vi "Read_MNK_Temperature.vi"(8 "Error in (no error)":errorcluster) -> (0 "Error out":errorcluster, 2 "Temperature (mK)":dbl)   [LabVIEW 2019, in "Inst.TC.MNK.lvclass"]
uses:
  Inst.TC.MNK.lvclass
  <userlib>/LevyLab/LV-Data/LV-Data.PG/API/Read Variable (double).vi
  <userlib>/LevyLab/LV-Data/LV-Data.PG/LV-Data.PGSQL.lvclass
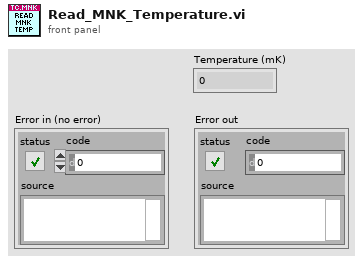
[diagram p1: front panel]
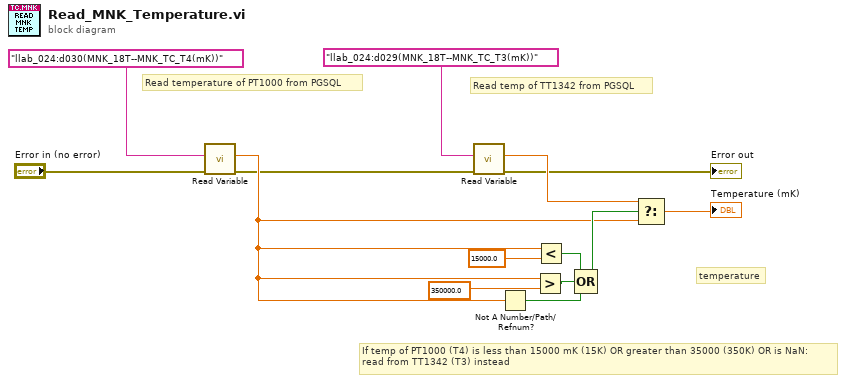
[diagram p0: block diagram]
diagram:
  # "If temp of PT1000 (T4) is less than 15000 mK (15K) OR greater than 35000 (350K) OR is NaN:\nread from TT1342 (T3) instead"
  # "Read temp of TT1342 from PGSQL"
  # "Read temperature of PT1000 from PGSQL"
  # "temperature"
  n1 = call-poly <userlib>:"Read Variable.vi"("error in (no error)"="Error in (no error)", "PG path"="llab_024:d030(MNK_18T--MNK_TC_T4(mK))") -> ("error out"=w3:errorcluster, "Value"=w6:dbl)  [unwired: 6 in, 2 out]
  n2 = call-poly <userlib>:"Read Variable.vi"("error in (no error)"=w3, "PG path"="llab_024:d029(MNK_18T--MNK_TC_T3(mK))") -> ("error out"=→"Error out":errorcluster, "Value"=w4:dbl)  [unwired: 6 in, 2 out]
  n3 = Not A Number/Path/Refnum?(number/path/refnum=w6) -> (NaN/Path/Refnum?=w11:bool)
  n4 = Greater?(x=w6, y=350000.0) -> (0:w9:bool)
  n5 = Less?(x=w6, y=15000.0) -> (x < y?=w12:bool)
  n6 = Compound Arithmetic op=OR(w12, w9, w11) -> (w10:bool)
  n7 = Select(t=w4, s=w10, f=w6) -> (s? t:f=→"Temperature (mK)":dbl)
